vi "Initialize.vi"(6 "active error checking":bool=TRUE, 8 "error in (no error)":errorcluster, 9 "reset":bool, 10 "ID query":bool=TRUE, 11 "VISA resource name":refnum<visa-resource-name>) -> (0 "error out":errorcluster, 3 "VISA resource name out":refnum<visa-resource-name>)   [LabVIEW 2016, in "Agilent 415X Series.lvlib"]
doc: "This VI establishes the communication with the instrument by querying the instrument for its ID string (optional via the front panel ID Query switch) and adding a new entry in the instrument table.\n\nThis VI also\n1. specifies whether to reset the instrument (optional)\n2. specifies whether to perform active error checking."
uses:
  Agilent 415X Series.lvlib
panel:
  # "(c) 2005-2015 National Instruments.  ALL RIGHTS RESERVED."
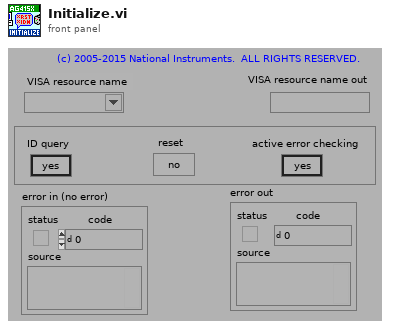
[diagram p1: front panel]
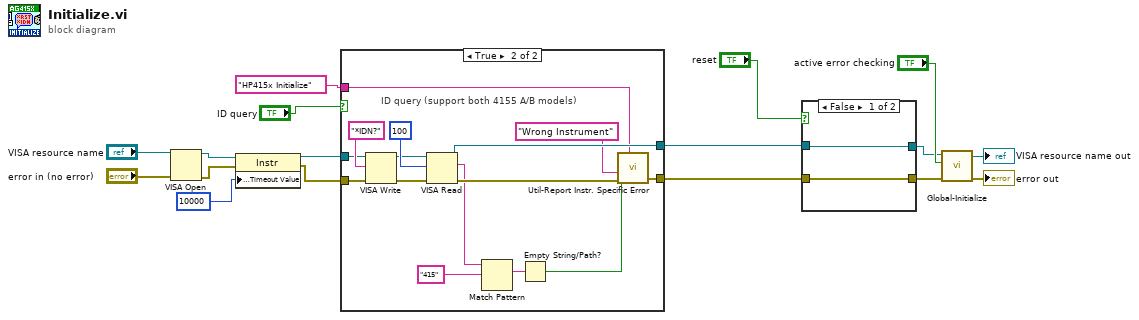
[diagram p0: block diagram]
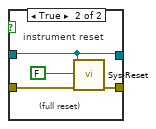
[diagram p2: hidden frame]
diagram:
  n1 = VISA Open(error in (no error)="error in (no error)", VISA resource name="VISA resource name") -> (VISA resource name=w2:refnum<visa-resource-name>, error out=w3:errorcluster)  [unwired: 3 in]
  n2 = property class="Instr"(reference=w2, error in=w3, "General Settings:Timeout Value"=u32 10000 ("Tmo Value")) -> (reference out=w7:refnum<visa-resource-name>, error out=w6:errorcluster)
  n3 = case shown="True" "ID query" {
    tunnel: w7 -> [w18 w30]
    tunnel: w6 -> [w19 w29]
    tunnel: [w19 w26] -> w15
    tunnel: [w18 w25] -> w16
    tunnel: "HP415x Initialize" ("VI name") -> [_ w24]
    frame False {
      # "no ID query"
    }
    frame True {
      # "ID query (support both 4155 A/B models)"
      n4 = VISA Write(VISA resource name=w30, write buffer="*IDN?", error in (no error)=w29) -> (VISA resource name out=w32:refnum<visa-resource-name>, error out=w31:errorcluster)  [unwired: 1 out]
      n5 = VISA Read(VISA resource name=w32, byte count=100, error in (no error)=w31) -> (VISA resource name out=w25:refnum<visa-resource-name>, read buffer=w22:string, error out=w27:errorcluster)  [unwired: 1 out]
      n6 = Match Pattern(string=w22, regular expression="415") -> (match substring=w21:string)  [unwired: 1 in, 3 out]
      n7 = Empty String/Path?(string/path=w21) -> (empty?=w20:bool)
      n8 = call "Util-Report Instr. Specific Error.vi"("source"=w24, "error in (no error)"=w27, "error message"="Wrong Instrument", "new error"=w20) -> ("error out"=w26:errorcluster)  [unwired: 6 in, 1 out]
    }
  }
  n9 = case shown="False" "reset" {
    tunnel: w16 -> [w36 w38]
    tunnel: w15 -> [w35 w39]
    tunnel: [w36 w38] -> w10
    tunnel: [w35 w40] -> w9
    frame False {
    }
    frame True {
      # "(full reset)"
      # "instrument reset"
      n10 = call "Sys-Reset.vi"("error in (no error)"=w39, "option"=FALSE, "VISA session"=w38) -> ("error out"=w40:errorcluster)  [unwired: 7 in, 1 out]
    }
  }
  n11 = call "Global-Initialize.vi"("error in (no error)"=w9, "active error checking"="active error checking", "VISA resource name"=w10) -> ("error out"=→"error out":errorcluster, "VISA resource name out"=→"VISA resource name out":refnum<visa-resource-name>)  [unwired: 7 in]
